vi "Save data.vi"(6 "Iteration index":i32, 7 "report in":refnum<class "NI_report.lvclass">, 8 "error in (no error)":errorcluster, 10 "DC readings":dbl[](array[numeric]), 11 "FFmeter settings in":T1={"AC Source"={"AC Source type"=enum."Fluke 5XXX calibrator", "VISA"="", "Ref. clock (Hz)"=0.0, "status ref"=refnum}, "TWM pipe"="", "Measurement status ref"=refnum, "TWM Status ref"=refnum, "Abort ref"=refnum, "DC meter"={"DC meter type"=enum."H/A/K 3458", "DC meter VISA"="", "NPLC"=0, "No of readings"=3, "status ref"=refnum}, "Measurement properties"={"Measurement frequencies (Hz)"=[], "Sampling frequency (Hz)"=0.0, "Signal amplitude (V)"=0.0, "AC-DC settle time (s)"=0.0, "Record length (multiples of period)"=[], "Measurement template file"=path "", "Row of START keyword"=0, "Row of STOP keyword"=0, "Calculate RMS from samples"=FALSE}} {"Measurement properties"."Record length (multiples of period)" format="%#_3p"; "Measurement properties"."Sampling frequency (Hz)" format="%#_3p"; "Measurement properties"."Measurement frequencies (Hz)" format="%#_3p"}) -> (0 "error out":errorcluster, 3 "FFmeter settings out":T1={"AC Source"={"AC Source type"=enum."Fluke 5XXX calibrator", "VISA"="", "Ref. clock (Hz)"=0.0, "status ref"=refnum}, "TWM pipe"="", "Measurement status ref"=refnum, "TWM Status ref"=refnum, "Abort ref"=refnum, "DC meter"={"DC meter type"=enum."H/A/K 3458", "DC meter VISA"="", "NPLC"=0, "No of readings"=3, "status ref"=refnum}, "Measurement properties"={"Measurement frequencies (Hz)"=[], "Sampling frequency (Hz)"=0.0, "Signal amplitude (V)"=0.0, "AC-DC settle time (s)"=0.0, "Record length (multiples of period)"=[], "Measurement template file"=path "", "Row of START keyword"=0, "Row of STOP keyword"=0, "Calculate RMS from samples"=FALSE}} {"Measurement properties"."Record length (multiples of period)" format="%#_3p"; "Measurement properties"."Sampling frequency (Hz)" format="%#_3p"; "Measurement properties"."Measurement frequencies (Hz)" format="%#_3p"}, 5 "report out":refnum<class "NI_report.lvclass">)   [LabVIEW 2020]
uses:
  GUI/Type definitions/FFmeter settings.ctl
  General AC source/Type definitions/AC Source.ctl
  General AC source/Type definitions/AC Source type.ctl
  General DC meter/Type definitions/DC meter.ctl
  General DC meter/Type definitions/DC meter type.ctl
  Measurement/Type definitions/Measuement properties.ctl
  <vilib>/Utility/NIReport.llb/NI_report.lvclass
  external libraries/varilib/varilib.lvlib
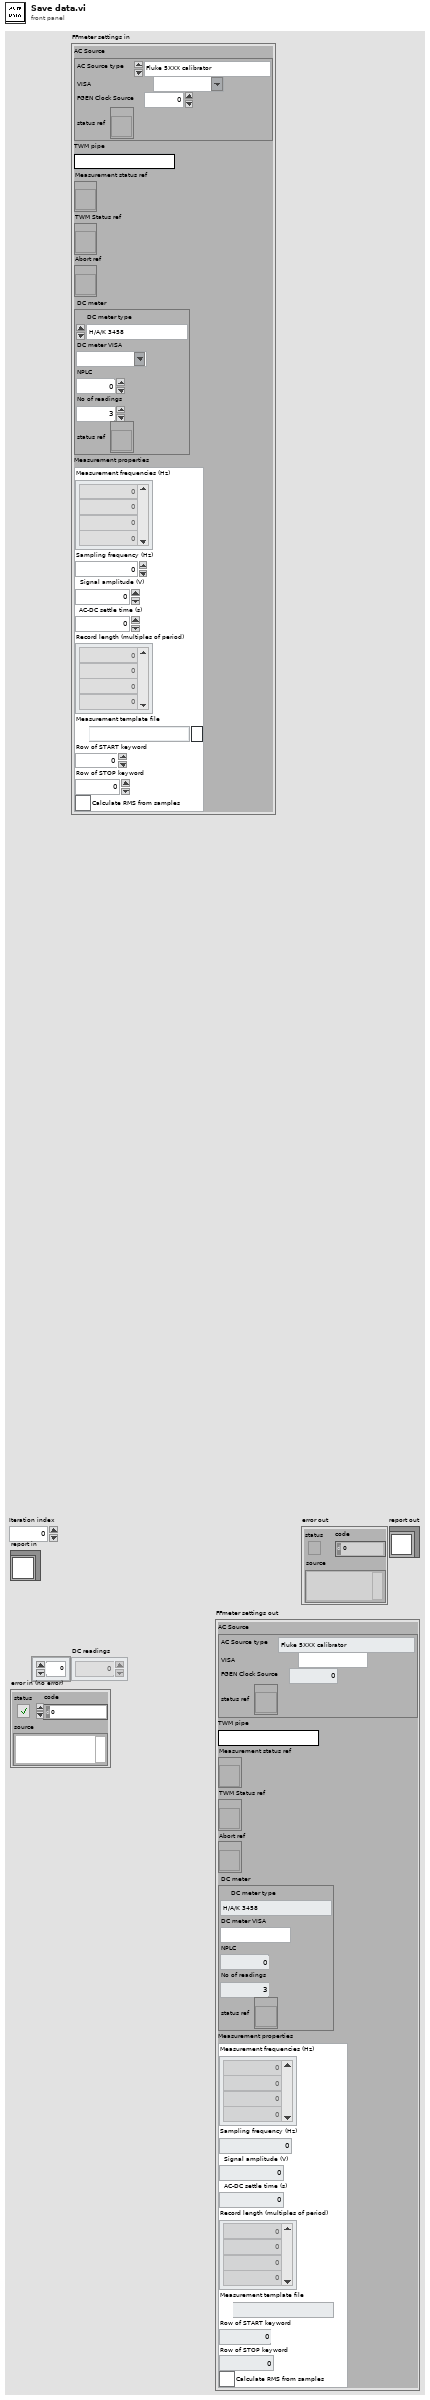
[diagram p1: front panel]
types:
  T1 = typedef "FFmeter settings.ctl" = cluster{"AC Source":T2, "TWM pipe":string, "Measurement status ref":refnum<vi>, "TWM Status ref":refnum<vi>, "Abort ref":refnum<vi>, "DC meter":T4, "Measurement properties":T6}
  T2 = typedef "AC Source.ctl" = cluster{"AC Source type":T3, "VISA":refnum<visa-resource-name>, "Ref. clock (Hz)":dbl, "status ref":refnum<vi>}
  T3 = typedef "AC Source type.ctl" = enum16{"Fluke 5XXX calibrator", "Tektronix AFG3101C", "dummy"}
  T4 = typedef "DC meter.ctl" = cluster{"DC meter type":T5, "DC meter VISA":refnum<visa-resource-name>, "NPLC":i32, "No of readings":i32, "status ref":refnum<vi>}
  T5 = typedef "DC meter type.ctl" = enum16{"H/A/K 3458", "FLuke 8508A", "dummy"}
  T6 = typedef "Measuement properties.ctl" = cluster{"Measurement frequencies (Hz)":dbl[], "Sampling frequency (Hz)":dbl, "Signal amplitude (V)":dbl, "AC-DC settle time (s)":dbl, "Record length (multiples of period)":dbl[], "Measurement template file":path, "Row of START keyword":i32, "Row of STOP keyword":i32, "Calculate RMS from samples":bool}
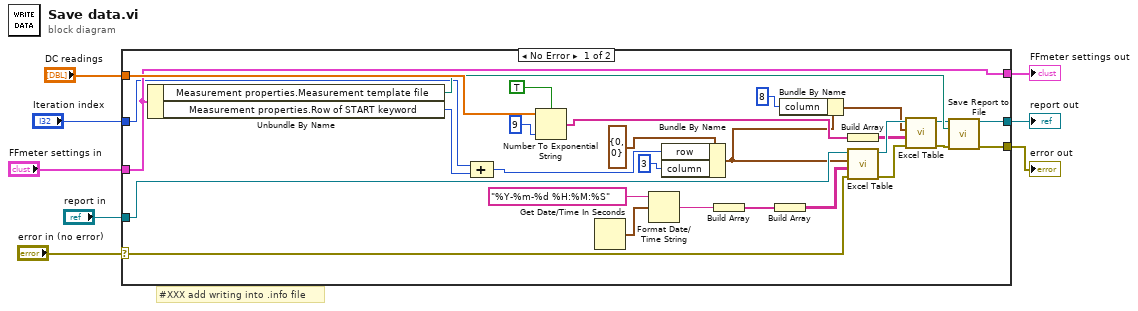
[diagram p0: block diagram]
diagram:
  # "#XXX add writing into .info file"
  n1 = case shown="No Error" "error in (no error)" {
    selector: "error in (no error)" -> [w21 w39]
    tunnel: "DC readings" -> [w36 _]
    tunnel: [w19 w39] -> w7
    tunnel: "FFmeter settings in" -> [w24 w38]
    tunnel: [w24 w38] -> w4
    tunnel: "Iteration index" -> [w22 _]
    tunnel: "report in" -> [w20 w37]
    tunnel: [w18 w37] -> w1
    frame No Error {
      n2 = Unbundle By Name(w24) -> ("Measurement properties.Measurement template file"=w23:path, "Measurement properties.Row of START keyword"=w27:i32)
      n3 = Compound Arithmetic op=ADD(w22, w27) -> (w28:i32)
      n4 = Number To Exponential String(number=w36, precision (6)=i16 9, 1:TRUE ("use system decimal point (T)")) -> (E-format string=w13:string[])  [unwired: 1 in]
      n5 = Get Date/Time In Seconds() -> (seconds since 1Jan1904=w29:timestamp)
      n6 = Format Date/Time String(time format string (%c)="%Y-%m-%d %H:%M:%S", seconds (now)=w29) -> (date/time string=w31:string)  [unwired: 1 in]
      n7 = Bundle By Name(cluster=cluster{"row":i32, "column":i32} {"row"=0, "column"=0} ("start (0, 0)"), "row"=w28, "column"=3) -> (w11:cluster{"row":i32, "column":i32})
      n8 = Build Array(w31) -> (w32:string[])
      n9 = Build Array(w32) -> (w33:string[][])
      n10 = Bundle By Name(cluster=w11, "column"=8) -> (w10:cluster{"row":i32, "column":i32})
      n11 = Build Array(w13) -> (w12:string[][])
      n12 = call "Excel Table.vi"("error in (no error)"=w21, "table"=w33, "start (0, 0)"=w11, "report in"=w20) -> ("error out"=w17:errorcluster, "report out"=w14:refnum<class "NI_report.lvclass">)  [unwired: 6 in]
      n13 = call "Excel Table.vi"("error in (no error)"=w17, "table"=w12, "start (0, 0)"=w10, "report in"=w14) -> ("error out"=w16:errorcluster, "report out"=w15:refnum<class "NI_report.lvclass">)  [unwired: 6 in]
      n14 = call-dynamic "Save Report to File.vi"("report in"=w15, "report file path"=w23, "error in (no error)"=w16) -> ("report out"=w18:refnum<class "NI_report.lvclass">, "error out"=w19:errorcluster)  [unwired: 11 in]
    }
    frame Error {
    }
  }
  "FFmeter settings out" <- w4
  "error out" <- w7
  "report out" <- w1
